vi "Get DBL EXPERIMENT.vi"(7 "Data Type (default value)":dbl, 9 "error in (no error)":errorcluster, 10 "Offset":i32, 11 "JSON":string) -> (1 "error out":errorcluster, 2 "Offset past match":i32, 3 "Number":dbl format="%.2f")   [LabVIEW 2015, in "JSONtext.lvlib"]
uses:
  JSONtext.lvlib
  String Subset.vi
  Advance past Number.vi
  Parsing Error.vi
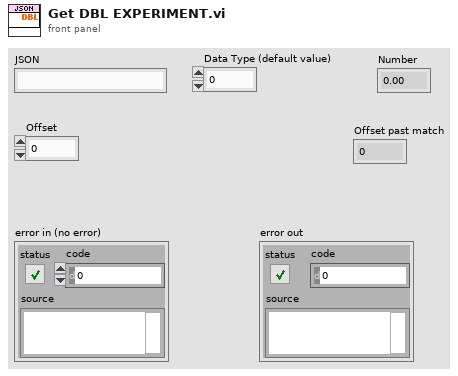
[diagram p1: front panel]
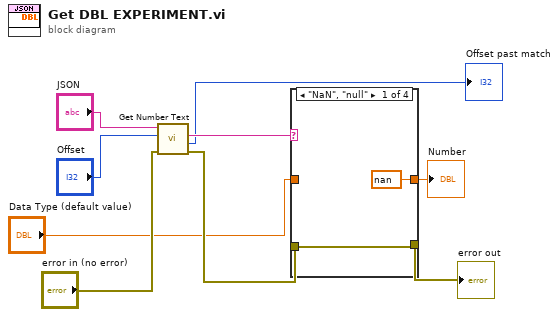
[diagram p0: block diagram]
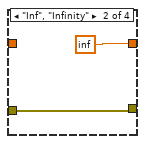
[diagram p2: hidden frame]
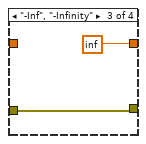
[diagram p3: hidden frame]
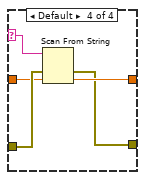
[diagram p4: hidden frame]
diagram:
  n1 = call "Get Number Text.vi"("error in (no error)"="error in (no error)", "Offset"="Offset", "JSON"="JSON") -> ("error out"=w6:errorcluster, "Offset past match"=→"Offset past match":i32, "Number Text"=w4:string)  [unwired: 6 in]
  n2 = case shown="\"NaN\", \"null\"" w4 {
    selector: w4 -> [_ _ _ w16]
    tunnel: [nan ("default value 1") inf ("default value 1") inf ("default value 1") w20] -> w3
    tunnel: w6 -> [w11 w12 w14 w19]
    tunnel: [w11 w12 w14 w18] -> w5
    tunnel: "Data Type (default value)" -> [_ _ _ w17]
    frame "NaN", "null" {
    }
    frame "Inf", "Infinity" {
    }
    frame "-Inf", "-Infinity" {
    }
    frame Default {
      n3 = Scan From String(input string=w16, error in=w19, default 1=w17) -> (error out=w18:errorcluster, output 1=w20:dbl)  [unwired: 2 in, 2 out]
    }
  }
  "error out" <- w5
  "Number" <- w3
